vi "GetAutomaticParameterMode.vi"(7 "Auto Parameter":T2, 8 "error in (no error)":errorcluster, 11 "Stream in":refnum<class "Stream.lvclass">) -> (0 "error out":errorcluster, 1 "Is Supported":bool, 2 "Automatic Parameter Mode":T1, 3 "Stream":refnum<class "Stream.lvclass">)   [LabVIEW 2020, in "capture.lvlib" / "Stream.lvclass"]
doc: "GetAutomaticParameterMode."
uses:
  Stream.lvclass
  Camera Automatic Parameters.ctl
  Camera Automatic Parameter Mode.ctl
  Stream.lvclass/Stream.ctl
  common/common.lvlib
  common/bin/gartoolkit_32-1.dll
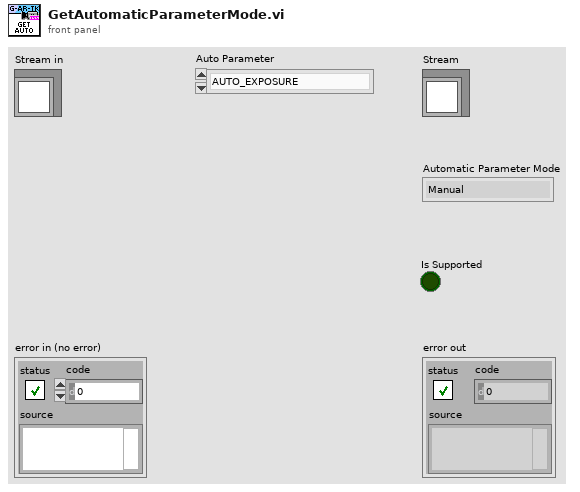
[diagram p1: front panel]
types:
  T1 = typedef "capture.lvlib/Stream.lvclass/Camera Automatic Parameter Mode.ctl" = enum16{"Manual", "Automatic"}
  T2 = typedef "capture.lvlib/Stream.lvclass/Camera Automatic Parameters.ctl" = enum16{"AUTO_EXPOSURE", "AUTO_FOCUS", "AUTO_WHITE_BALANCE", "AUTO_GAIN"}
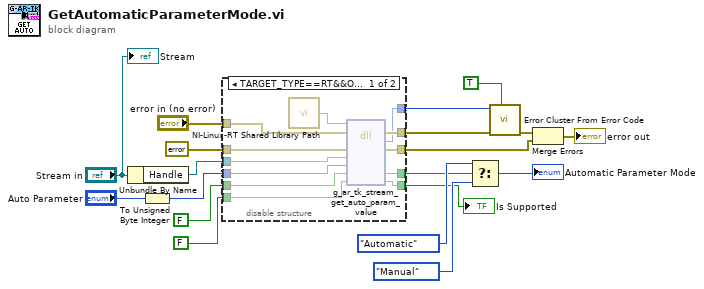
[diagram p0: block diagram]
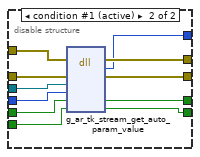
[diagram p2: hidden frame]
diagram:
  n1 = Unbundle By Name("Stream in") -> ("Handle"=w10:refnum<data-value>)
  n2 = To Unsigned Byte Integer(number="Auto Parameter") -> (unsigned 8bit integer=w9:u8)
  n3 = disable-structure shown="TARGET_TYPE==RT&&OS==Linux" {
    disable-tunnel: "error in (no error)" -> [w30 w42]
    disable-tunnel: errorcluster {"status"=FALSE, "code"=0, "source"=""} ("error constant") -> [w29 w41]
    disable-tunnel: w10 -> [w28 w40]
    disable-tunnel: w9 -> [w27 w39]
    disable-tunnel: FALSE -> [w26 w38]
    disable-tunnel: FALSE -> [w25 w37]
    disable-tunnel: [w24 w36] -> w6
    disable-tunnel: [w23 w35] -> w5
    disable-tunnel: [w22 w34] -> w4
    disable-tunnel: [w21 w33] -> w3
    disable-tunnel: [w20 w32] -> w2
    frame condition #0 {
      n4 = call "NI-Linux-RT Shared Library Path.vi"() -> ("Path"=w31:path)
      n5 = dll-call lib="?" fn="g_ar_tk_stream_get_auto_param_value" ("g_ar_toolkit.*.*:g_ar_tk_stream_capture_next")(path in=w31, error in=w30, "error_cluster"=w29, "EDVR_strm"=w28, "parameter"=w27, "is_automatic"=w26, "is_supported"=w25) -> (error out=w24:errorcluster, "MgErr"=w23:i32, "error_cluster"=w22:errorcluster, "is_automatic"=w21:bool, "is_supported"=w20:bool)  [unwired: 3 in, 1 out]
    }
    frame condition #1 (active) {
      n6 = dll-call lib="C:/serenial/lib/g-augmented-reality-toolkit/LabVIEW/common/bin/gartoolkit_*-1.*" fn="g_ar_tk_stream_get_auto_param_value" ("g_ar_toolkit.*.*:g_ar_tk_stream_capture_next")(error in=w42, "error_cluster"=w41, "EDVR_strm"=w40, "parameter"=w39, "is_automatic"=w38, "is_supported"=w37) -> (error out=w36:errorcluster, "MgErr"=w35:i32, "error_cluster"=w34:errorcluster, "is_automatic"=w33:bool, "is_supported"=w32:bool)  [unwired: 4 in, 1 out]
    }
  }
  "Is Supported" <- w2
  n7 = Select(t=Camera_Automatic_Parameter_Mode."Automatic" ("Automatic Parameter Mode"), s=w3, f=Camera_Automatic_Parameter_Mode."Manual") -> (s? t:f=→"Automatic Parameter Mode":T1)
  n8 = call <vilib>:"Error Cluster From Error Code.vi"("show call chain? (False)"=TRUE, "error in (no error)"=w6, "error code (0)"=w5) -> ("error out"=w16:errorcluster)  [unwired: 6 in]
  n9 = Merge Errors(w16, w4) -> (→"error out":errorcluster)
  "Stream" <- "Stream in"
